vi "action.vi"(0 "HGF_Device_IDN":refnum<class "HGF_Device_IDN.lvclass">, 2 "HGF_Visitable":refnum<class "HGF_Visitable.lvclass">, 5 "error in (no error)":errorcluster) -> (14 "dup HGF_Device_IDN":refnum<class "HGF_Device_IDN.lvclass">, 16 "dup HGF_Visitable":refnum<class "HGF_Visitable.lvclass">, 19 "error out":errorcluster)   [LabVIEW 2014, in "HGF_DeviceBaseClasses.lvlib" / "HGF_Device_IDN.lvclass"]
doc: "This is a dynamic dispatch VI that is called from Visitor.visit(). It will call member VIs of Visitable to perform the requested action which means: calling public methods of Visitable child class.\n\n<B>Hint:</B> This method is abstract and need to be implemented by child classes."
uses:
  HGF_Device_IDN.lvclass
  HGF_DeviceBase/HGF_DeviceBase.lvclass
  HGF_BaseClasses/HGF_Visitable/HGF_Visitable.lvclass
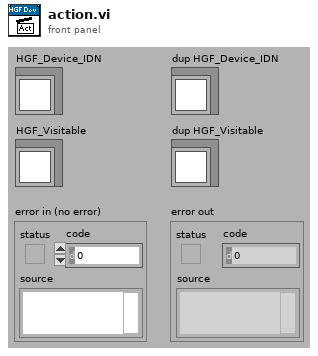
[diagram p1: front panel]
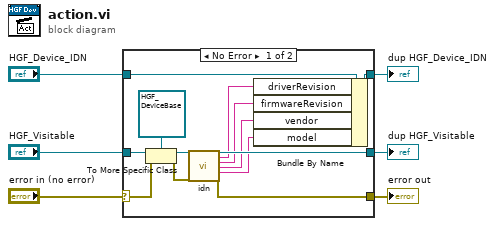
[diagram p0: block diagram]
diagram:
  n1 = case shown="No Error" "error in (no error)" {
    selector: "error in (no error)" -> [w17 w21]
    tunnel: "HGF_Visitable" -> [w19 w22]
    tunnel: [w13 w22] -> w5
    tunnel: [w8 w21] -> w3
    tunnel: [w15 w20] -> w1
    tunnel: "HGF_Device_IDN" -> [w16 w20]
    frame No Error {
      n2 = To More Specific Class(target class=refnum<class "HGF_DeviceBase.lvclass"> refnum ("HGF_DeviceBaseClasses.lvlib:HGF_DeviceBase.lvclass"), reference=w19, error in=w17) -> (specific class reference=w14:refnum<class "HGF_DeviceBase.lvclass">, error out=w7:errorcluster)
      n3 = call "idn.vi"("HGF_DeviceBase"=w14, "error in (no error)"=w7) -> ("dup HGF_DeviceBase"=w13:refnum<class "HGF_DeviceBase.lvclass">, "driverRevision"=w12:string, "firmwareRevision"=w11:string, "vendor"=w10:string, "model"=w9:string, "error out"=w8:errorcluster)  [unwired: 12 out]
      n4 = Bundle By Name(cluster=w16, "driverRevision"=w12, "firmwareRevision"=w11, "vendor"=w10, "model"=w9) -> (w15:refnum<class "HGF_Device_IDN.lvclass">)
    }
    frame Error {
    }
  }
  "error out" <- w3
  "dup HGF_Device_IDN" <- w1
  "dup HGF_Visitable" <- w5
